vi "zeemanlockmonitor.vi"(0 "error in":errorcluster) -> (1 "Zeeman out of lock?":bool, 3 "error out":errorcluster)   [LabVIEW 2013]
doc: "This VI alerts the user if the Verdi laser is overheating. The VI polls a voltage output from Barium that is +5V if the Verdi is overheating and 0V otherwise. Assuming the monitoring VI is running on Barium, this should alert the otherwise unsuspecting operator that the Verdi is having issues."
uses:
  <vilib>/DAQmx/read.llb/DAQmx Read (Analog DBL 1Chan 1Samp).vi
  <vilib>/DAQmx/miscellaneous.llb/DAQmx Fill In Error Info.vi
panel:
  out "0 V indicates out of lock.":dbl=1.7484243024816801 format="%0.2f"
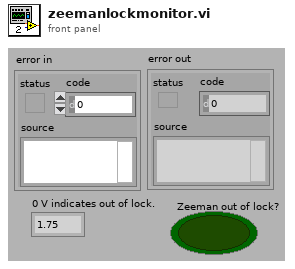
[diagram p1: front panel]
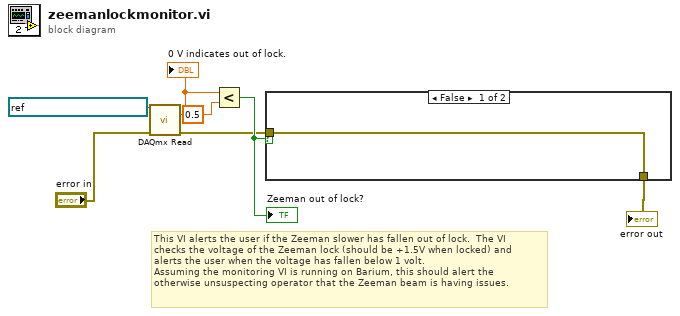
[diagram p0: block diagram]
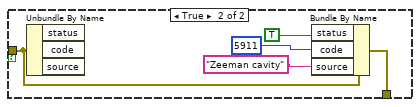
[diagram p2: hidden frame]
diagram:
  # "This VI alerts the user if the Zeeman slower has fallen out of lock.  The VI\nchecks the voltage of the Zeeman lock (should be +1.5V when locked) and\nalerts the user when the voltage has fallen below 1 volt. \nAssuming the monitoring VI is running on Barium, this should alert the\notherwise unsuspecting operator that the Zeeman beam is having issues."
  n1 = call-poly <vilib>:"DAQmx Read.vi"("task/channels in"=refnum<k21> "ZeemanLockMonitor", "error in"="error in") -> ("data"=w4:dbl, "error out"=w2:errorcluster)  [unwired: 11 in, 1 out]
  "0 V indicates out of lock." <- w4
  n2 = Less?(x=w4, y=0.5 ("x")) -> (x < y?=w3:bool)
  "Zeeman out of lock?" <- w3
  n3 = case shown="False" w3 {
    tunnel: w2 -> [w8 w13]
    tunnel: [w8 w11] -> w1
    frame False {
    }
    frame True {
      n4 = Unbundle By Name(w13) -> ()  [unwired: 3 out]
      n5 = Bundle By Name(cluster=w13, "status"=TRUE, "code"=5911, "source"="Zeeman cavity" ("message")) -> (w11:errorcluster)
    }
  }
  "error out" <- w1
